vi "Sequences to Bytes.vi"(10 "Channel states":bool[][](array[boolean])=[[FALSE, FALSE, FALSE, FALSE, FALSE, FALSE, FALSE, FALSE, FALSE, FALSE, FALSE, FALSE], [TRUE, FALSE, FALSE, FALSE, FALSE, FALSE, FALSE, FALSE, FALSE, FALSE, FALSE, FALSE], [TRUE, TRUE, FALSE, FALSE, FALSE, FALSE, FALSE, FALSE, FALSE, FALSE, FALSE, FALSE], [TRUE, TRUE, TRUE, TRUE, TRUE, TRUE, TRUE, FALSE, FALSE, FALSE, FALSE, FALSE], [TRUE, TRUE, TRUE, TRUE, TRUE, TRUE, TRUE, TRUE, FALSE, FALSE, FALSE, FALSE], [TRUE, TRUE, TRUE, TRUE, TRUE, TRUE, TRUE, TRUE, TRUE, FALSE, FALSE, FALSE], [TRUE, TRUE, TRUE, TRUE, TRUE, TRUE, TRUE, TRUE, TRUE, TRUE, TRUE, FALSE], [TRUE, TRUE, TRUE, TRUE, TRUE, TRUE, TRUE, TRUE, TRUE, TRUE, TRUE, TRUE]]) -> (1 "Ch. bytes 2":u8[](array[numeric]), 2 "Ch. bytes 1":u8[](array[numeric]))   [LabVIEW 2020, in "QuPMXdriver.lvlib"]
doc: "Converts sequences (array of channel states) to bytes."
uses:
  QuPMXdriver.lvlib
panel:
  out "channels":i32
  out "states":i32
  out "Number of channels":i32
  out "Aux":i8
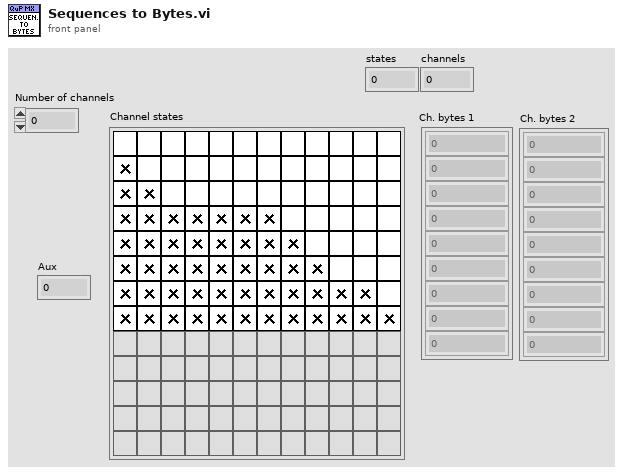
[diagram p1: front panel]
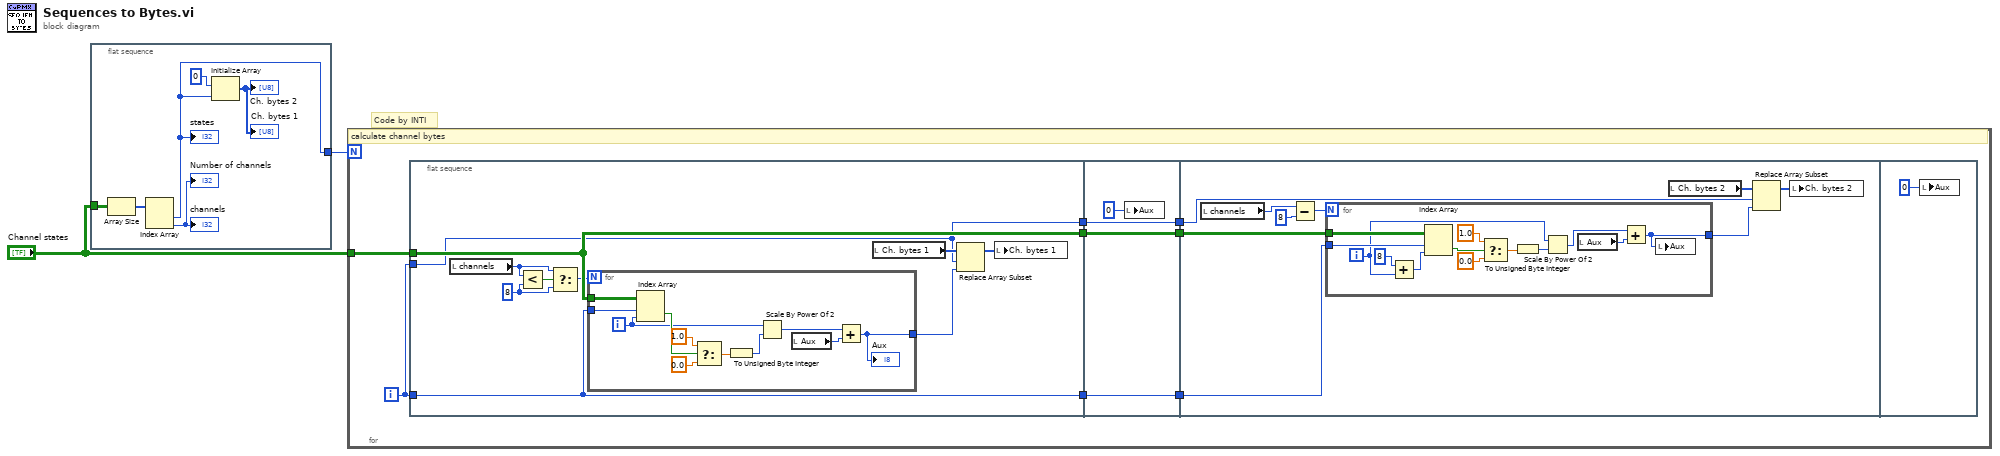
[diagram p0: block diagram]
diagram:
  # "Code by INTI"
  n1 = flat-sequence {
    tunnel: [w4] -> w2
    tunnel: "Channel states" -> [w5]
    frame #0 {
      n2 = Array Size(array=w5) -> (size(s)=w6:i32[])
      n3 = Index Array(array=w6) -> (element #1=w4:i32, element #2=→"Number of channels" →"channels":i32)  [unwired: 2 in]
      "states" <- w4
      n4 = Initialize Array(0, w4) -> (→"Ch. bytes 1" →"Ch. bytes 2":i32[])
    }
  }
  n5 = for {
    N: w2 -> [_]
    tunnel: "Channel states" -> [w16]
    i -> [w15]
    # "calculate channel bytes"
    n6 = flat-sequence {
      tunnel: w16 -> [w26]
      tunnel: [w26] -> w14
      tunnel: w15 -> [w25]
      tunnel: [w25] -> w13
      tunnel: w15 -> [w21]
      tunnel: [w21] -> w12
      tunnel: w14 -> [w40]
      tunnel: [w40] -> w11
      tunnel: w13 -> [w39]
      tunnel: [w39] -> w10
      tunnel: w12 -> [w38]
      tunnel: [w38] -> w9
      tunnel: w11 -> [w50]
      tunnel: w10 -> [w49]
      tunnel: w9 -> [w44]
      frame #0 {
        w17 = 8 ("y")
        n7 = local read "channels"() -> (w18:i32)
        n8 = Less?(x=w18, y=w17) -> (x < y?=w24:bool)
        n9 = Select(t=w18, s=w24, f=w17) -> (s? t:f=w23:i32)
        n10 = for {
          N: w23 -> [_]
          tunnel: w26 -> [w37]
          tunnel: w25 -> [w30]
          tunnel: [w29] -> w20
          i -> [w32]
          n11 = Index Array(array=w37, index (row)=w30, index (col)=w32) -> (element=w36:bool)
          n12 = Select(t=1.0, s=w36, f=0.0) -> (s? t:f=w27:dbl)
          n13 = To Unsigned Byte Integer(number=w27) -> (unsigned 8bit integer=w28:u8)
          n14 = Scale By Power Of 2(n=w32, x=w28) -> (x*2^n=w33:u8)
          n15 = local read "Aux"() -> (w31:i8)
          n16 = Add(x=w33, y=w31) -> (x+y=w29:u8)
          "Aux" <- w29
        }
        n17 = local read "Ch. bytes 1"() -> (w22:u8[])
        n18 = Replace Array Subset(array=w22, new element=w20, index=w21) -> (w19:u8[])
        n19 = local write "Ch. bytes 1"(w19) -> ()
      }
      frame #1 {
        n20 = local write "Aux"(i8 0 ("Aux")) -> ()
      }
      frame #2 {
        n21 = local read "channels"() -> (w47:i32)
        n22 = Subtract(x=w47, y=8) -> (x-y=w48:i32)
        n23 = for {
          N: w48 -> [_]
          tunnel: w50 -> [w63]
          tunnel: w49 -> [w57]
          tunnel: [w53] -> w42
          i -> [w54]
          n24 = Add(x=8, y=w54) -> (x+y=w55:i32)
          n25 = Index Array(array=w63, index (row)=w57, index (col)=w55) -> (element=w62:bool)
          n26 = Select(t=1.0, s=w62, f=0.0) -> (s? t:f=w52:dbl)
          n27 = To Unsigned Byte Integer(number=w52) -> (unsigned 8bit integer=w51:u8)
          n28 = Scale By Power Of 2(n=w54, x=w51) -> (x*2^n=w59:u8)
          n29 = local read "Aux"() -> (w58:i8)
          n30 = Add(x=w59, y=w58) -> (x+y=w53:u8)
          n31 = local write "Aux"(w53) -> ()
        }
        n32 = local read "Ch. bytes 2"() -> (w45:u8[])
        n33 = Replace Array Subset(array=w45, new element=w42, index=w44) -> (w43:u8[])
        n34 = local write "Ch. bytes 2"(w43) -> ()
      }
      frame #3 {
        n35 = local write "Aux"(i8 0 ("Aux")) -> ()
      }
    }
  }
